vi "controlRealtimeInputLoopMode.vi"(7 "Set":bool, 8 "error in":errorcluster, 9 "RT Loop in":i32, 10 "axis in":u8, 11 "connection ID":i32) -> (0 "error out":errorcluster, 1 "RT Loop out":i32, 2 "axis out":u8, 3 "connection ID":i32)   [LabVIEW 2016]
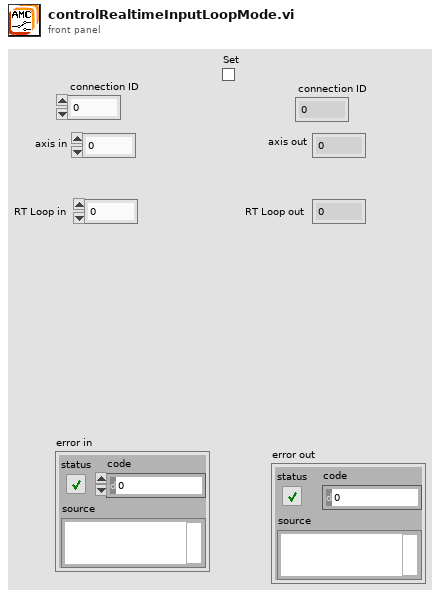
[diagram p1: front panel]
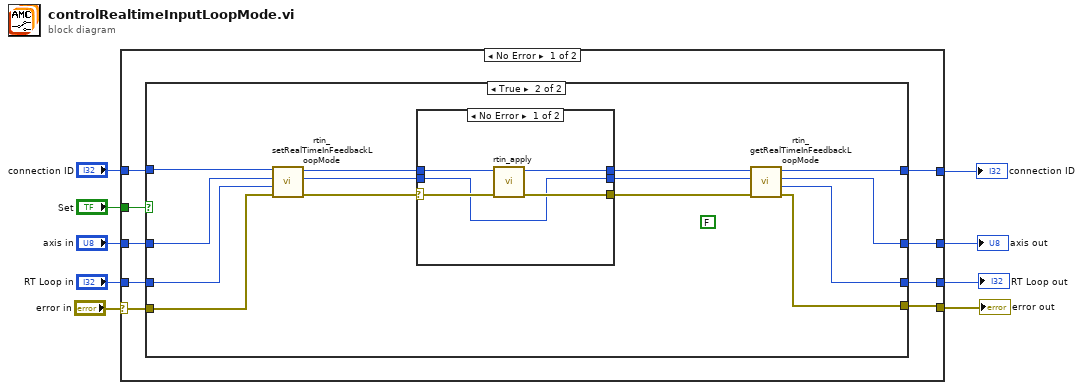
[diagram p0: block diagram]
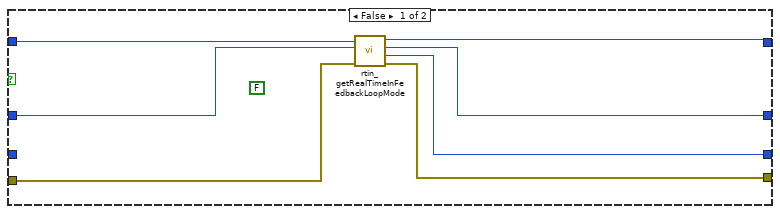
[diagram p2: hidden frame]
diagram:
  n1 = case shown="No Error" "error in" {
    selector: "error in" -> [w12 w51]
    tunnel: "axis in" -> [w16 w49]
    tunnel: [w13 w51] -> w8
    tunnel: [w11 w49] -> w7
    tunnel: "Set" -> [w17 _]
    tunnel: [w14 w48] -> w5
    tunnel: "connection ID" -> [w18 w48]
    tunnel: "RT Loop in" -> [w15 w50]
    tunnel: [w10 w50] -> w2
    frame No Error {
      n2 = case shown="True" w17 {
        tunnel: [w24 w31] -> w14
        tunnel: w18 -> [w25 w39]
        tunnel: w16 -> [w21 w37]
        tunnel: [w22 w29] -> w13
        tunnel: w15 -> [_ w35]
        tunnel: w12 -> [w23 w34]
        tunnel: [w20 w27] -> w11
        tunnel: [w19 w28] -> w10
        frame False {
          (unwired) FALSE ("tempvalue")
          n3 = call "rtin_getRealTimeInFeedbackLoopMode.vi"("error in"=w23, "axis"=w21, "connection ID"=w25) -> ("error out"=w22:errorcluster, "mode"=w19:i32, "axis_out"=w20:i32, "connection ID"=w24:i32)  [unwired: 5 in]
        }
        frame True {
          (unwired) FALSE ("tempvalue")
          n4 = call "rtin_setRealTimeInFeedbackLoopMode.vi"("error in"=w34, "mode"=w35, "axis"=w37, "connection ID"=w39) -> ("error out"=w33:errorcluster, "axis_out"=w36:i32, "connection ID"=w38:i32)  [unwired: 5 in]
          n5 = case shown="No Error" w33 {
            selector: w33 -> [w42 w47]
            tunnel: [w41 w47] -> w30
            tunnel: w38 -> [w44 w46]
            tunnel: [w43 w46] -> w32
            tunnel: w36 -> [w40 w45]
            tunnel: [w40 w45] -> w26
            frame No Error {
              n6 = call "rtin_apply.vi"("error in"=w42, "connection ID"=w44) -> ("error out"=w41:errorcluster, "connection ID"=w43:i32)  [unwired: 8 in]
            }
            frame Error {
            }
          }
          n7 = call "rtin_getRealTimeInFeedbackLoopMode.vi"("error in"=w30, "axis"=w26, "connection ID"=w32) -> ("error out"=w29:errorcluster, "mode"=w28:i32, "axis_out"=w27:i32, "connection ID"=w31:i32)  [unwired: 5 in]
        }
      }
    }
    frame Error {
    }
  }
  "error out" <- w8
  "axis out" <- w7
  "connection ID" <- w5
  "RT Loop out" <- w2
